vi "TestPointer.Clear Error.vi"   [LabVIEW 2016, in "TestPointer.lvclass"]
uses:
  TestPointer.lvclass
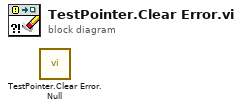
[diagram p0: block diagram]
diagram:
  n1 = call "TestPointer.Clear Error.Null.vi"() -> ()  [unwired: 10 in, 2 out]
